vi "whilep loop.vi"() -> ()   [LabVIEW 2013]
panel:
  in  "Boolean 3":bool
  out "Tank 3":dbl(slide) scale=0.0..1000.0
  out "Numeric 3":dbl
  in  "valor 3":dbl
  out "Tank 2":dbl(slide) scale=0.0..1000.0
  out "Numeric 2":dbl
  in  "valor 2":dbl
  in  "Boolean":bool
  out "Boolean 2":bool
  out "Tank":dbl(slide) scale=0.0..1000.0
  out "Numeric":dbl
  in  "valor":dbl
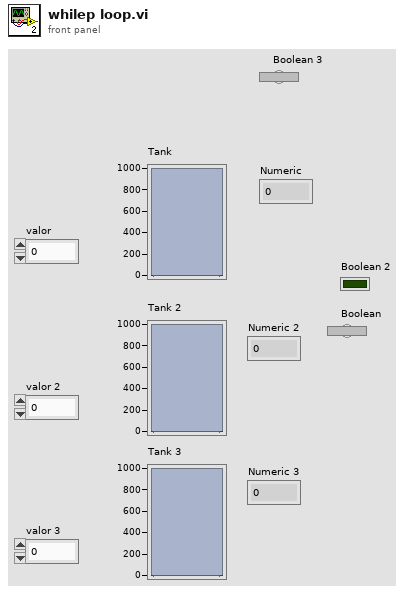
[diagram p1: front panel]
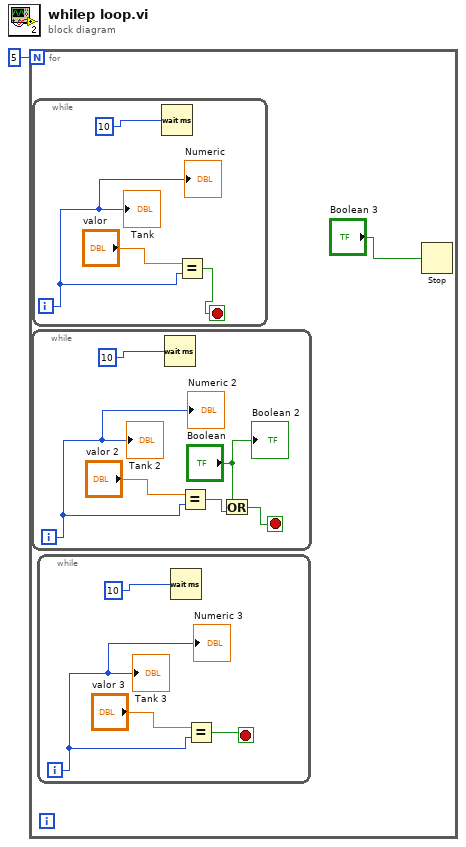
[diagram p0: block diagram]
diagram:
  n1 = for {
    N: 5 -> [_]
    n2 = while {
      i -> [w10]
      stop <- w8 stop-if-true
      n3 = Wait (ms)(milliseconds to wait=u32 10 ("millisecond timer value")) -> ()  [unwired: 1 out]
      n4 = Equal?(x="valor 2", y=w10) -> (x = y?=w9:bool)
      n5 = Or(x="Boolean", y=w9) -> (x .or. y?=w8:bool)
      "Tank 2" <- w10
      "Numeric 2" <- w10
      "Boolean 2" <- "Boolean"
    }
    n6 = while {
      i -> [w14]
      stop <- w13 stop-if-true
      n7 = Wait (ms)(milliseconds to wait=u32 10 ("millisecond timer value")) -> ()  [unwired: 1 out]
      n8 = Equal?(x="valor", y=w14) -> (x = y?=w13:bool)
      "Tank" <- w14
      "Numeric" <- w14
    }
    n9 = while {
      i -> [w4]
      stop <- w3 stop-if-true
      n10 = Wait (ms)(milliseconds to wait=u32 10 ("millisecond timer value")) -> ()  [unwired: 1 out]
      n11 = Equal?(x="valor 3", y=w4) -> (x = y?=w3:bool)
      "Tank 3" <- w4
      "Numeric 3" <- w4
    }
    n12 = Stop(stop? (T)="Boolean 3") -> ()
  }
